vi "5. SCADA_Robotic_Arm_1.vi"() -> ()   [LabVIEW 2019]
panel:
  in  "Tab Control":enum32{"Control Panel"}(tab)
  in  "Bottle Pic":bool
  in  "Slider":dbl(slide) scale=157.0..420.0
  out "Boolean":bool
  out "Boolean 4":bool
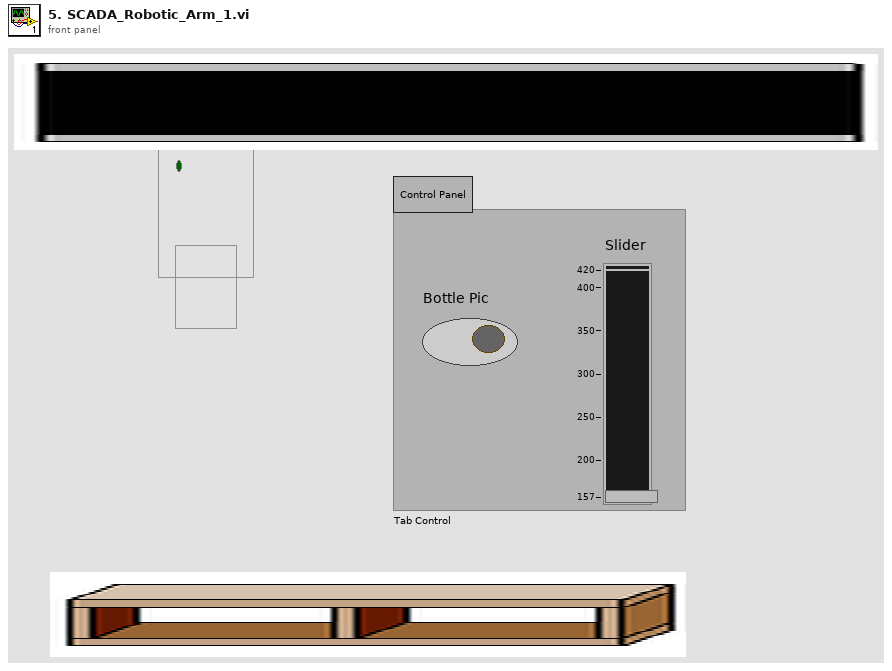
[diagram p1: front panel]
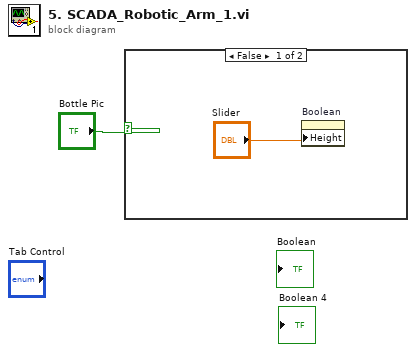
[diagram p0: block diagram]
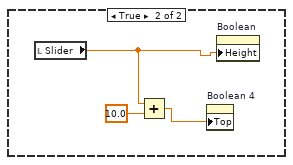
[diagram p2: hidden frame]
diagram:
  n1 = case shown="False" "Bottle Pic" {
    frame False {
      n2 = property on="Boolean" class="Bool (strict)"("Height"="Slider") -> ()  [unwired: 2 in, 2 out]
    }
    frame True {
      n3 = local read "Slider"() -> (w5:dbl)
      n4 = Add(x=w5, y=10.0) -> (x+y=w4:dbl)
      n5 = property on="Boolean 4" class="Bool (strict)"("Top"=w4) -> ()  [unwired: 2 in, 2 out]
      n6 = property on="Boolean" class="Bool (strict)"("Height"=w5) -> ()  [unwired: 2 in, 2 out]
    }
  }
